vi "onLinkageErrors.vi"(8 "error in (no error)":errorcluster, 11 "Test Runner in":refnum<class "Test Runner.lvclass">) -> (0 "error out":errorcluster, 3 "Test Runner out":refnum<class "Test Runner.lvclass">)   [LabVIEW 2020, in "Caraya.lvlib" / "Test Runner.lvclass"]
uses:
  Test Runner.lvclass
  Test Runner.lvclass/Test Runner.ctl
  Assert/Assert Not Error.vi
  Test/Test.lvclass
  Assert/Assert.lvclass
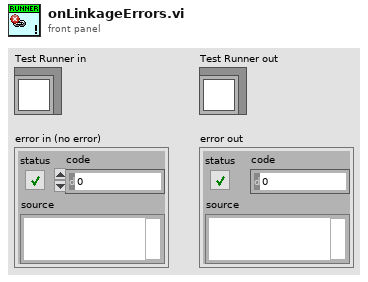
[diagram p1: front panel]
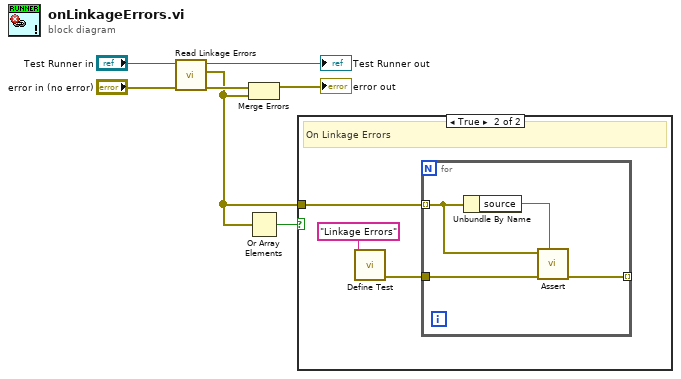
[diagram p0: block diagram]
diagram:
  n1 = call "Read Linkage Errors.vi"("error in (no error)"="error in (no error)", "Test Runner in"="Test Runner in") -> ("error out"=w6:errorcluster, "Linkage Errors"=w2:errorcluster[], "Test Runner out"=→"Test Runner out":refnum<class "Test Runner.lvclass">)  [unwired: 7 in]
  n2 = Merge Errors(w6, w2) -> (→"error out":errorcluster)
  n3 = Or Array Elements(Boolean array=w2) -> (logical OR=w1:bool)
  n4 = case shown="True" w1 {
    tunnel: w2 -> [_ w8]
    frame False {
      # "No Linkage Errors"
    }
    frame True {
      # "On Linkage Errors"
      n5 = call "Define Test.vi"("Label (VI Title)"="Linkage Errors" ("Label")) -> ("error out"=w9:errorcluster)  [unwired: 9 in, 1 out]
      n6 = for {
        tunnel: w9 -> [w14]
        tunnel: [w13] -> _ mode=indexing
        tunnel: w8 -> [w12] mode=indexing
        n7 = Unbundle By Name(w12) -> ("source"=w11:string)
        n8 = call-poly "Assert.vi"("Label"=w11, "error in (no error)"=w14, "Not Error?"=w12) -> ("error out"=w13:errorcluster)  [unwired: 7 in, 1 out]
      }
    }
  }
